vi "connect.vi"(2 "error in":errorcluster, 3 "VISA resource name":refnum<visa-resource-name>) -> (0 "error out":errorcluster, 1 "VISA resource name out":refnum<visa-resource-name>)   [LabVIEW 2014, in "stepper3D.lvlib"]
doc: "Use this template to build a VI to use as a subVI."
uses:
  <vilib>/Instr/_visa.llb/VISA Configure Serial Port (Instr).vi
  stepper3D.lvlib
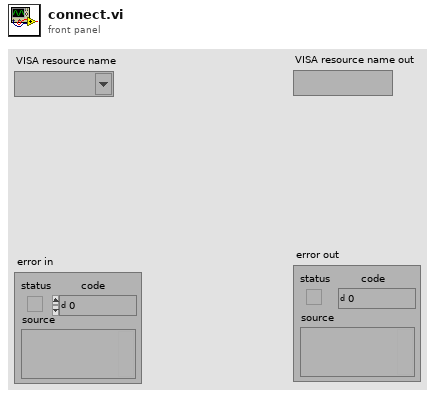
[diagram p1: front panel]
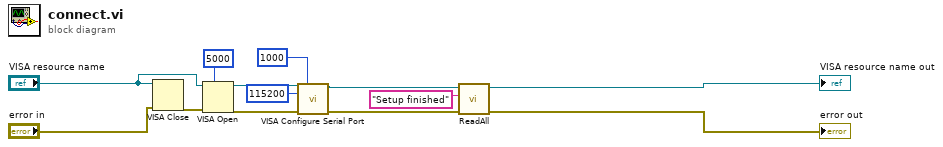
[diagram p0: block diagram]
diagram:
  n1 = VISA Close(VISA resource name="VISA resource name", error in (no error)="error in") -> (error out=w7:errorcluster)
  n2 = VISA Open(timeout (0)=u32 5000 ("VISA Open timeout (0)"), error in (no error)=w7, VISA resource name="VISA resource name") -> (VISA resource name=w12:refnum<visa-resource-name>, error out=w10:errorcluster)  [unwired: 2 in]
  n3 = call-poly "VISA Configure Serial Port"("VISA resource name"=w12, "timeout (10sec)"=u32 1000, "baud rate (9600)"=u32 115200, "error in (no error)"=w10) -> ("VISA resource name out"=w9:refnum<visa-resource-name>, "error out"=w8:errorcluster)  [unwired: 10 in]
  n4 = call "ReadAll.vi"("error in (no error)"=w8, "value"="Setup finished", "VISA resource in"=w9) -> ("error out"=→"error out":errorcluster, "VISA resource out"=→"VISA resource name out":refnum<visa-resource-name>)  [unwired: 5 in, 2 out]
